vi "EllipseOverlay.vi"(9 "Fitted Parameters (Pixel)":dbl[](array[numeric])) -> (2 "Array":cluster{"x out":dbl, "y out":dbl}[](array[cluster]))   [LabVIEW 2015]
uses:
  <vilib>/Analysis/coordinate.llb/2D Cartesian Coordinate Rotation (Scalar).vi
  <vilib>/Analysis/NI_AALPro.lvlib
panel:
  out "Center y":dbl
  out "Center x":dbl
  in  "Number of Points":u16=100
  out "theta (degree)":dbl
  out "Width B":dbl
  out "Width A":dbl
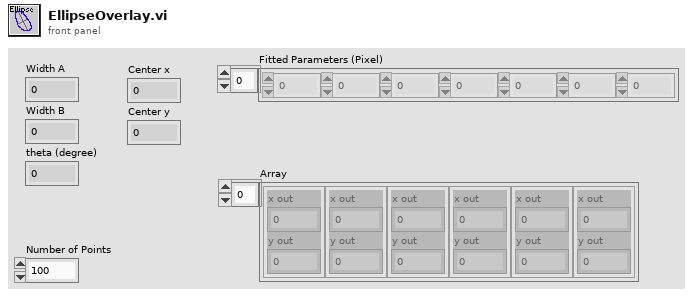
[diagram p1: front panel]
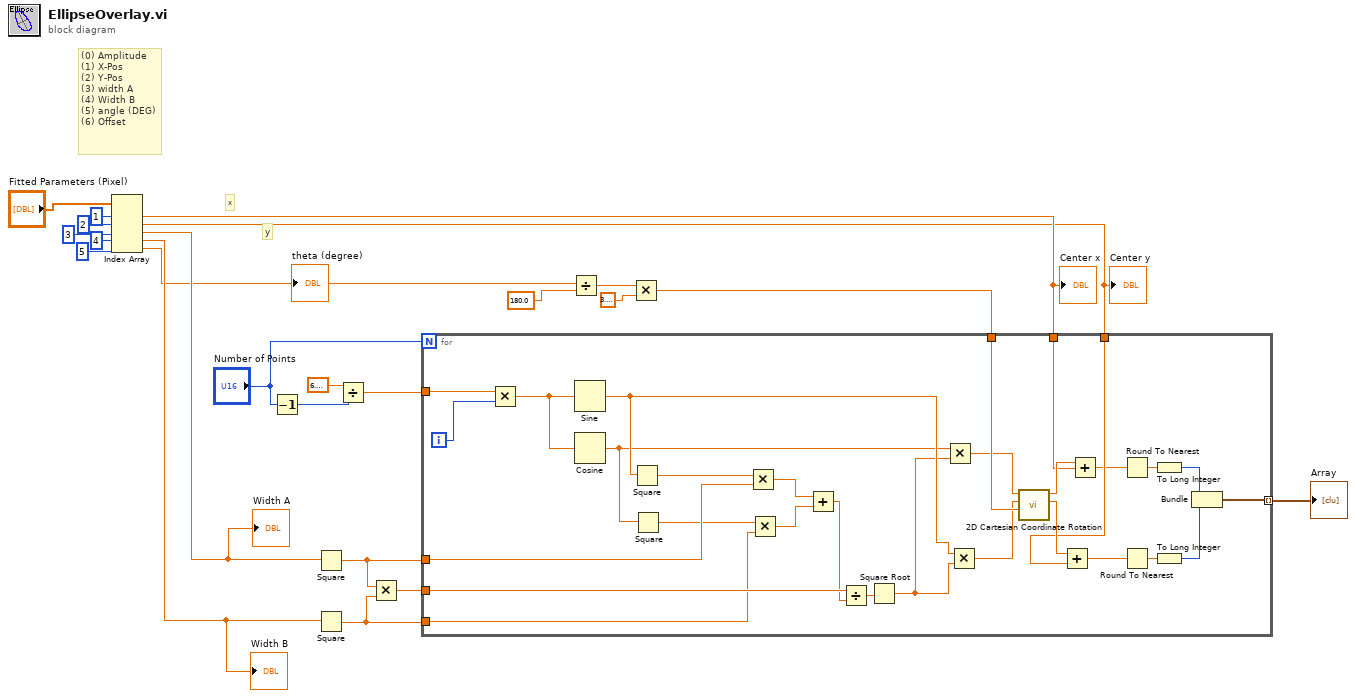
[diagram p0: block diagram]
diagram:
  # "y"
  # "x"
  # "(0) Amplitude\n(1) X-Pos\n(2) Y-Pos\n(3) width A\n(4) Width B\n(5) angle (DEG)\n(6) Offset"
  n1 = Index Array(array="Fitted Parameters (Pixel)", index #1=1 ("index"), index #2=2 ("index"), index #3=3 ("index"), index #4=4 ("index"), index #5=5 ("index")) -> (element #1=w5:dbl, element #2=w4:dbl, element #3=w3:dbl, element #4=w2:dbl, element #5=w1:dbl)
  "Width A" <- w3
  "Width B" <- w2
  "theta (degree)" <- w1
  "Center x" <- w5
  "Center y" <- w4
  n2 = Decrement(x="Number of Points") -> (x-1=w22:u16)
  n3 = Square(x=w3) -> (x^2=w19:dbl)
  n4 = Square(x=w2) -> (x^2=w18:dbl)
  n5 = Divide(x=6.283185307179586, y=w22) -> (x/y=w21:dbl)
  n6 = Multiply(x=w19, y=w18) -> (x*y=w20:dbl)
  n7 = Divide(x=w1, y=180.0) -> (x/y=w15:dbl)
  n8 = Multiply(x=w15, y=3.141592653589793) -> (x*y=w14:dbl)
  n9 = for {
    N: "Number of Points" -> [_]
    tunnel: w21 -> [w50]
    tunnel: w20 -> [w49]
    tunnel: w19 -> [w45]
    tunnel: w18 -> [w44]
    tunnel: [w37] -> w16 mode=indexing
    tunnel: w14 -> [w36]
    tunnel: w5 -> [w31]
    tunnel: w4 -> [w30]
    i -> [w38]
    n10 = Multiply(x=w50, y=w38) -> (x*y=w51:dbl)
    n11 = Sine(x=w51) -> (sin(x)=w48:dbl)
    n12 = Cosine(x=w51) -> (cos(x)=w47:dbl)
    n13 = Square(x=w48) -> (x^2=w46:dbl)
    n14 = Square(x=w47) -> (x^2=w43:dbl)
    n15 = Multiply(x=w46, y=w45) -> (x*y=w42:dbl)
    n16 = Multiply(x=w43, y=w44) -> (x*y=w41:dbl)
    n17 = Add(x=w42, y=w41) -> (x+y=w40:dbl)
    n18 = Divide(x=w49, y=w40) -> (x/y=w52:dbl)
    n19 = Square Root(x=w52) -> (sqrt(x)=w39:dbl)
    n20 = Multiply(x=w47, y=w39) -> (x*y=w35:dbl)
    n21 = Multiply(x=w48, y=w39) -> (x*y=w34:dbl)
    n22 = call-poly <vilib>:"2D Cartesian Coordinate Rotation.vi"("theta"=w36, "y"=w34, "x"=w35) -> ("y out"=w32:dbl, "x out"=w33:dbl)  [unwired: 6 in, 1 out]
    n23 = Add(x=w32, y=w30) -> (x+y=w25:dbl)
    n24 = Add(x=w33, y=w31) -> (x+y=w27:dbl)
    n25 = Round To Nearest(number=w27) -> (nearest integer value=w26:dbl)
    n26 = Round To Nearest(number=w25) -> (nearest integer value=w24:dbl)
    n27 = To Long Integer(number=w26) -> (32bit integer=w29:i32)
    n28 = To Long Integer(number=w24) -> (32bit integer=w28:i32)
    n29 = Bundle(w29, w28) -> (w37:cluster{i32, i32})  [unwired: 1 in]
  }
  "Array" <- w16
